vi "IronsWindFunction.vi"(9 "Desired Irons Angle":dbl, 10 "Angle to test":dbl) -> (2 "Goodness":dbl)   [LabVIEW 2011]
uses:
  2 Classes/LinearInterpolation/LinearInterpolation.lvclass
  2 Typedefs/apparent wind direction.ctl
  2 Globals/2 Global.vi
  2 Globals/2 TuningConstants.vi
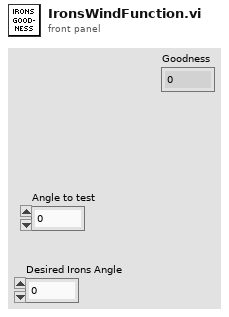
[diagram p1: front panel]
types:
  T1 = typedef "absolute wind direction.ctl" = dbl
  T2 = typedef "apparent wind direction.ctl" = dbl
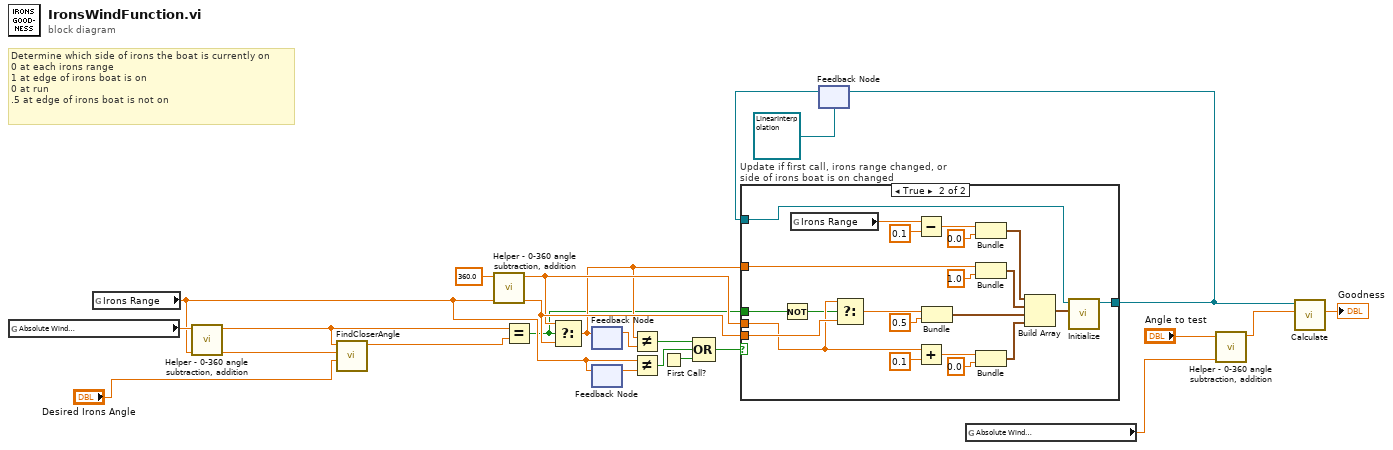
[diagram p0: block diagram]
diagram:
  # "Determine which side of irons the boat is currently on\n0 at each irons range\n1 at edge of irons boat is on\n0 at run\n.5 at edge of irons boat is not on"
  n1 = global read "2 Global.vi" "Absolute Wind\nDirection (º)"() -> (w24:T1)
  n2 = global read "2 TuningConstants.vi" "Irons Range"() -> (w16:dbl)
  n3 = call "Helper - 0-360 angle subtraction, addition.vi"("y"=w16, "x"=w24) -> ("x + y"=w23:dbl, "x - y"=w19:T2)  [unwired: 8 in]
  n4 = call "FindCloserAngle.vi"("Central Angle"="Desired Irons Angle", "Angle 2"=w23, "Angle 1"=w19) -> ("Closer Angle"=w20:T2)  [unwired: 8 in]
  n5 = call "Helper - 0-360 angle subtraction, addition.vi"("y"=w16, "x"=360.0) -> ("x + y"=w21:dbl, "x - y"=w18:T2)  [unwired: 8 in]
  n6 = Equal?(x=w19, y=w20) -> (x = y?=w6:bool)
  n7 = Select(t=w18, s=w6, f=w21) -> (s? t:f=w14:T2)
  n8 = feedback-in #1(w14) -> ()
  n9 = feedback #1() -> (w15:T2)  [unwired: 1 in]
  n10 = feedback-in #2(w16) -> ()
  n11 = feedback #2() -> (w17:dbl)  [unwired: 1 in]
  n12 = Not Equal?(x=w14, y=w15) -> (x != y?=w11:bool)
  n13 = Not Equal?(x=w16, y=w17) -> (x != y?=w12:bool)
  n14 = First Call?() -> (First Call?: T/F=w13:bool)
  n15 = Compound Arithmetic op=OR(w11, w12, w13) -> (w10:bool)
  n16 = feedback #3(refnum<class "LinearInterpolation.lvclass"> refnum ("LinearInterpolation out")) -> (w7:refnum<class "LinearInterpolation.lvclass">)
  n17 = case "Update if first call, irons range changed, or  side of irons boat is on changed" shown="True" w10 {
    tunnel: [w25 w47] -> w9
    tunnel: w14 -> [_ w42]
    tunnel: w6 -> [_ w26]
    tunnel: w21 -> [_ w41]
    tunnel: w18 -> [_ w34]
    tunnel: w7 -> [w25 w28]
    frame False {
    }
    frame True {
      n18 = Not(x=w26) -> (.not. x?=w27:bool)
      n19 = global read "2 TuningConstants.vi" "Irons Range"() -> (w38:dbl)
      n20 = Select(t=w34, s=w27, f=w41) -> (s? t:f=w40:T2)
      n21 = Subtract(x=w38, y=0.1) -> (x-y=w36:dbl)
      n22 = Add(x=w34, y=T2 0.1) -> (x+y=w32:T2)
      n23 = Bundle("x - y"=w40, "Closer Angle"=T2 0.5) -> (w43:cluster{"x - y":T2, "Closer Angle":T2})  [unwired: 1 in]
      n24 = Bundle(w36, "Closer Angle"=T2 0.0) -> (w35:cluster{dbl, "Closer Angle":T2})  [unwired: 1 in]
      n25 = Bundle("x - y"=w42, "Closer Angle"=T2 1.0) -> (w45:cluster{"x - y":T2, "Closer Angle":T2})  [unwired: 1 in]
      n26 = Bundle("x - y"=w32, "Closer Angle"=T2 0.0) -> (w30:cluster{"x - y":T2, "Closer Angle":T2})  [unwired: 1 in]
      n27 = Build Array(w35, w45, w43, w30) -> (w29:cluster{"x - y":T2, "Closer Angle":T2}[])
      n28 = call "Initialize.vi"("Angle-Value Pairs"=w29, "LinearInterpolation in"=w28) -> ("LinearInterpolation out"=w47:refnum<class "LinearInterpolation.lvclass">)  [unwired: 8 in, 1 out]
    }
  }
  n29 = feedback-in #3(w9) -> ()
  n30 = global read "2 Global.vi" "Absolute Wind\nDirection (º)"() -> (w3:T1)
  n31 = call "Helper - 0-360 angle subtraction, addition.vi"("y"=w3, "x"="Angle to test") -> ("x - y"=w2:T2)  [unwired: 8 in, 1 out]
  n32 = call-dynamic "Calculate.vi"("X (degrees)"=w2, "AngleFunction in"=w9) -> ("AngleFunction(X)"=→"Goodness":dbl)  [unwired: 7 in, 2 out]
